vi "Robot Global Data.vi"() -> ()   [LabVIEW 2012]
doc: "This global VI can contain as many global variables as you need. Place a control on the panel, give it a good name. To read or write to it from a VI, drag the icon to the diagram of that VI. You can also drag from the project. Click on the node to change which global you access. You shouldn't have multiple locations writing to a global or it will cause a race-condition."
uses:
  <vilib>/Rock Robotics/WPI/Camera/WPI_CameraImageSize.ctl
  BasketType.ctl
panel:
  in  "LauncherSteerControl":bool
  in  "AutoCenter":bool
  in  "BoundingBox":T1
  in  "MaxRPM":dbl=1350.0
  in  "SetMaxRPM":bool
  in  "UpCloseRPMReverse":dbl=690.0
  in  "SetUpCloseRPM":bool
  in  "KeyRPM":dbl=935.0
  in  "UpCloseRPM":dbl=653.0
  in  "SelectIndex":dbl
  in  "SelectedIndex":dbl
  in  "Target Index":dbl
  out "Target Info Legacy":T2(array[cluster])
  in  "FireReverse":bool
  in  "Selected Target":T3
  in  "Target Info":T4(array[cluster])
  in  "ArmControl":dbl
  in  "ArmActuateReverse":bool
  in  "LauncherSpeedR":dbl
  in  "Enable CamServo":bool
  in  "Autonomous":bool
  in  "UseRobotGyro":bool
  in  "ArmRollerReverse":bool
  in  "Fire":bool
  in  "Aim Angle Error":dbl
  out "Aim: OK to Shoot?":bool
  in  "LeftRightBasket":dbl
  in  "TopBottomBasket":dbl
  in  "ArmRoller":bool
  in  "Ball Collector Reverse":bool
  in  "Set RPM":dbl
  in  "LauncherSpeed":dbl
  in  "ReadDriveEncoders":bool
  in  "DriveDistance":dbl
  in  "Brake":bool
  in  "RobotGyro":dbl
  in  "Basket":T5=enum."Top"
  in  "LauncherPower":dbl(slide) scale=1.0..-1.0
  in  "LauncherSteer":dbl(slide) scale=-1.0..1.0
  in  "TankDriveRight":dbl(slide) scale=1.0..-1.0
  in  "RunLauncher":bool
  in  "StraightDrive":bool
  in  "Ball Collector":bool
  in  "SpeedControl":bool
  in  "EnableAim":bool=TRUE
  in  "ArmActuate":bool
  in  "TankDriveLeft":dbl(slide) scale=1.0..-1.0
  in  "TargetDistance":dbl
  in  "LauncherGyro":dbl
  in  "UseLauncherGyro":bool
  in  "LED toggle rate (ms)":u32=20
  in  "image size":T6
  in  "Enable Vision":bool
  # "DRIVER"
  # "SHOOTER"
  # "DANGEROUS"
  # "Originally 684.8"
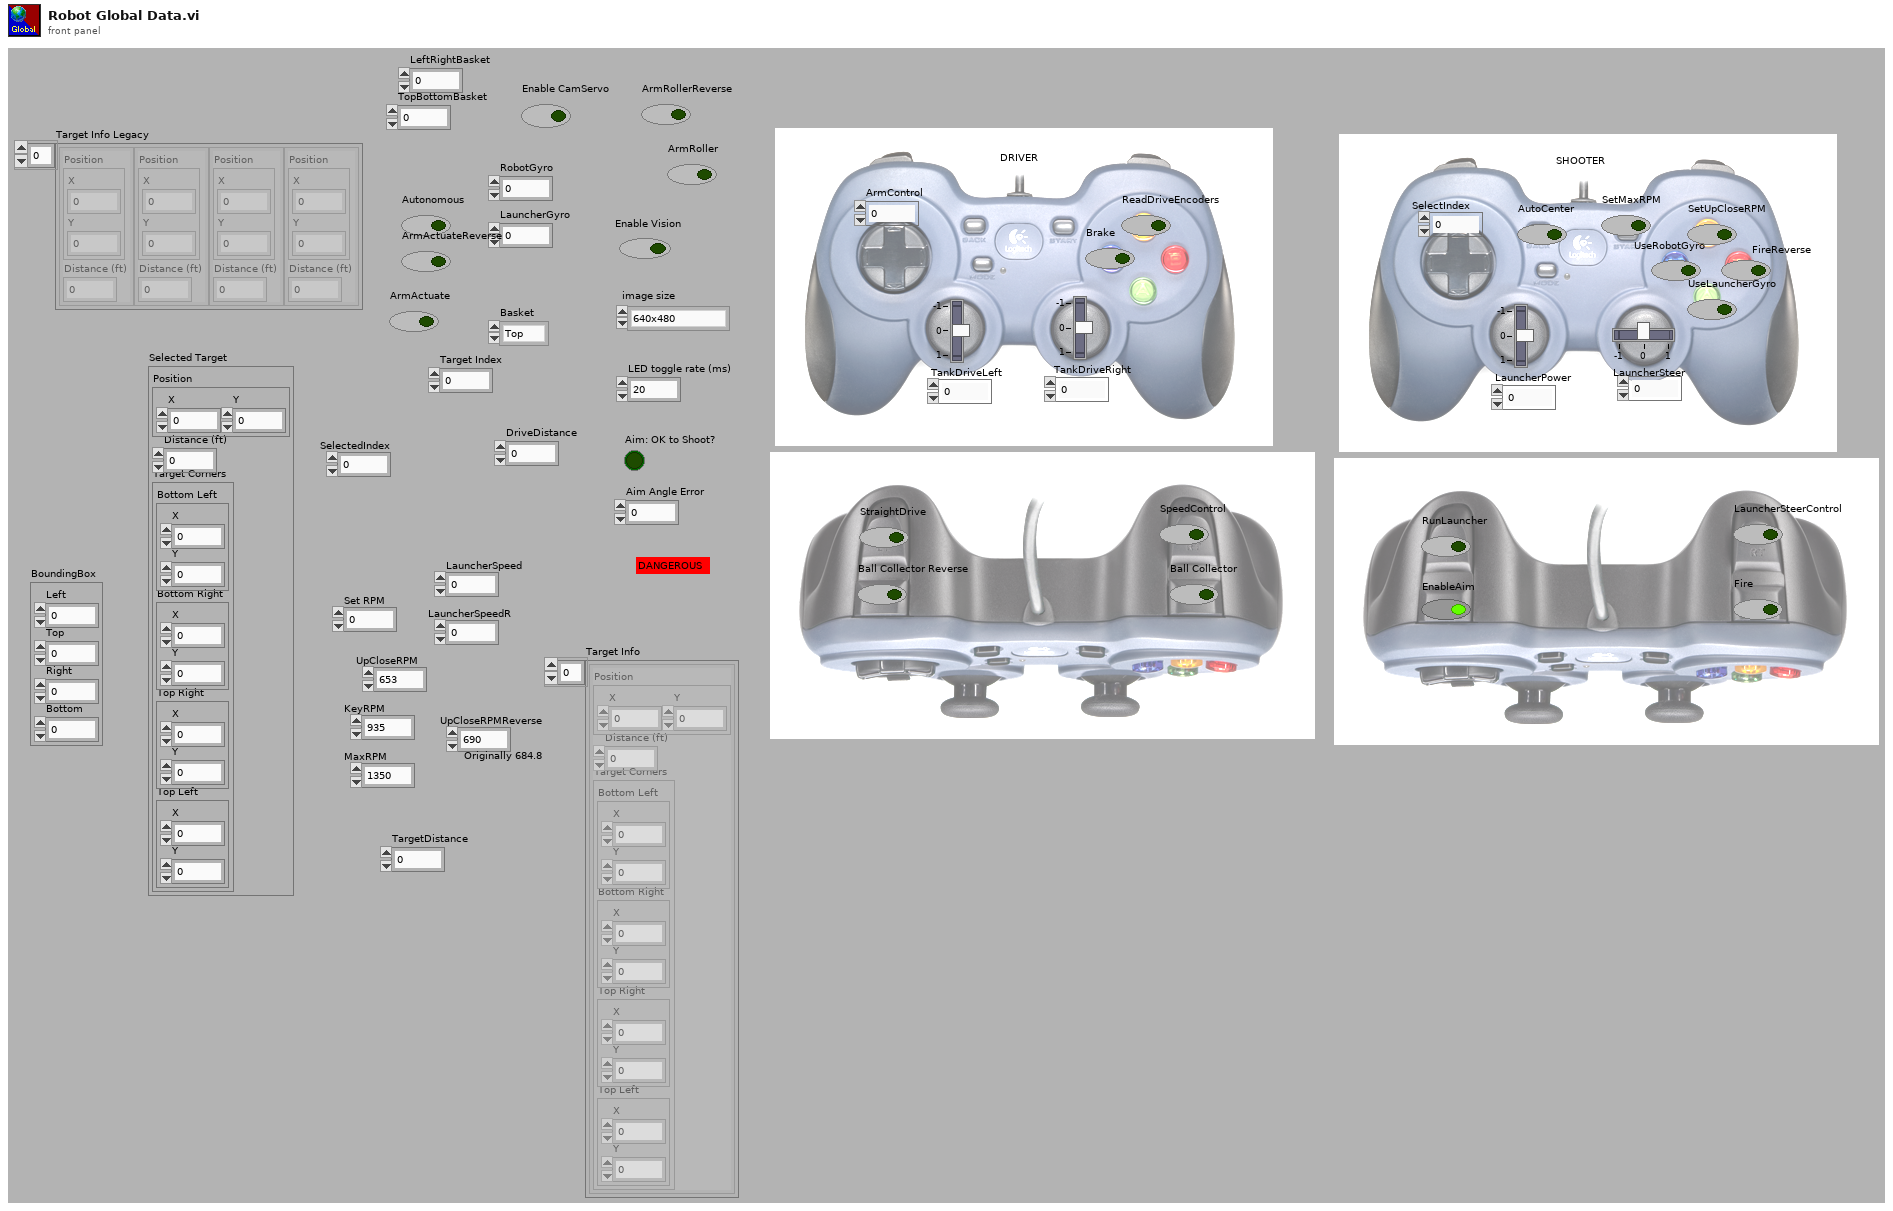
[diagram p1: front panel]
types:
  T1 = cluster{"Left":dbl, "Top":dbl, "Right":dbl, "Bottom":dbl}
  T2 = cluster{"Position":cluster{"X":dbl, "Y":dbl}, "Distance (ft)":dbl}[]
  T3 = cluster{"Position":cluster{"X":dbl, "Y":dbl}, "Distance (ft)":dbl, "Target Corners":cluster{"Bottom Left":cluster{"X":dbl, "Y":dbl}, "Bottom Right":cluster{"X":dbl, "Y":dbl}, "Top Right":cluster{"X":dbl, "Y":dbl}, "Top Left":cluster{"X":dbl, "Y":dbl}}}
  T4 = cluster{"Position":cluster{"X":dbl, "Y":dbl}, "Distance (ft)":dbl, "Target Corners":cluster{"Bottom Left":cluster{"X":dbl, "Y":dbl}, "Bottom Right":cluster{"X":dbl, "Y":dbl}, "Top Right":cluster{"X":dbl, "Y":dbl}, "Top Left":cluster{"X":dbl, "Y":dbl}}}[]
  T5 = typedef "BasketType.ctl" = enum16{"Left", "Bottom", "Right", "Top"}
  T6 = typedef "WPI_CameraImageSize.ctl" = enum16{"640x480", "320x240", "160x120"}
diagram:
